vi "Project_G18.vi"() -> ()   [LabVIEW 2022 SP3]
uses:
  <vilib>/DAQmx/read.llb/DAQmx Read (Digital Bool 1Line 1Point).vi
  <vilib>/DAQmx/read.llb/DAQmx Read (Analog 1D DBL NChan 1Samp).vi
  <vilib>/DAQmx/create/channels.llb/DAQmx Create Channel (DI-Digital Input).vi
  <vilib>/DAQmx/create/channels.llb/DAQmx Create Channel (AI-Voltage-Basic).vi
  <vilib>/DAQmx/miscellaneous.llb/DAQmx Fill In Error Info.vi
panel:
  out "BIN STATUS:":string
  out "Dry Waste":bool
  in  "VISA resource name 3":refnum<visa-resource-name>
  in  "Numeric Controller":dbl
  in  "VISA resource name 6":refnum<visa-resource-name>
  out "Object Detector":bool
  in  "Object detector line":tag
  in  "physical channels":tag
  out "Fill level of the bin":u8(slide) scale=0.0..10.0
  out "Wet Waste":bool
  out "Numeric":dbl
  out "Wet/Dry Meter":dbl(knob) scale=0.0..10.0
  in  "Metal detector line":tag
  out "Metal Detector":bool
  in  "VISA resource name 2":refnum<visa-resource-name>
  in  "VISA resource name":refnum<visa-resource-name>
  in  "stop":bool
  # "Smart Waste Management System"
  # "WET"
  # "DRY"
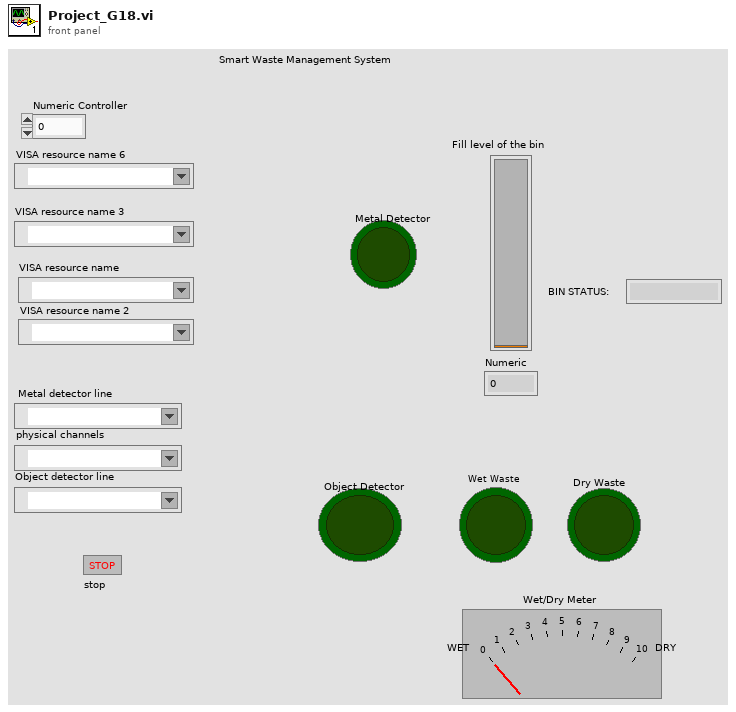
[diagram p1: front panel]
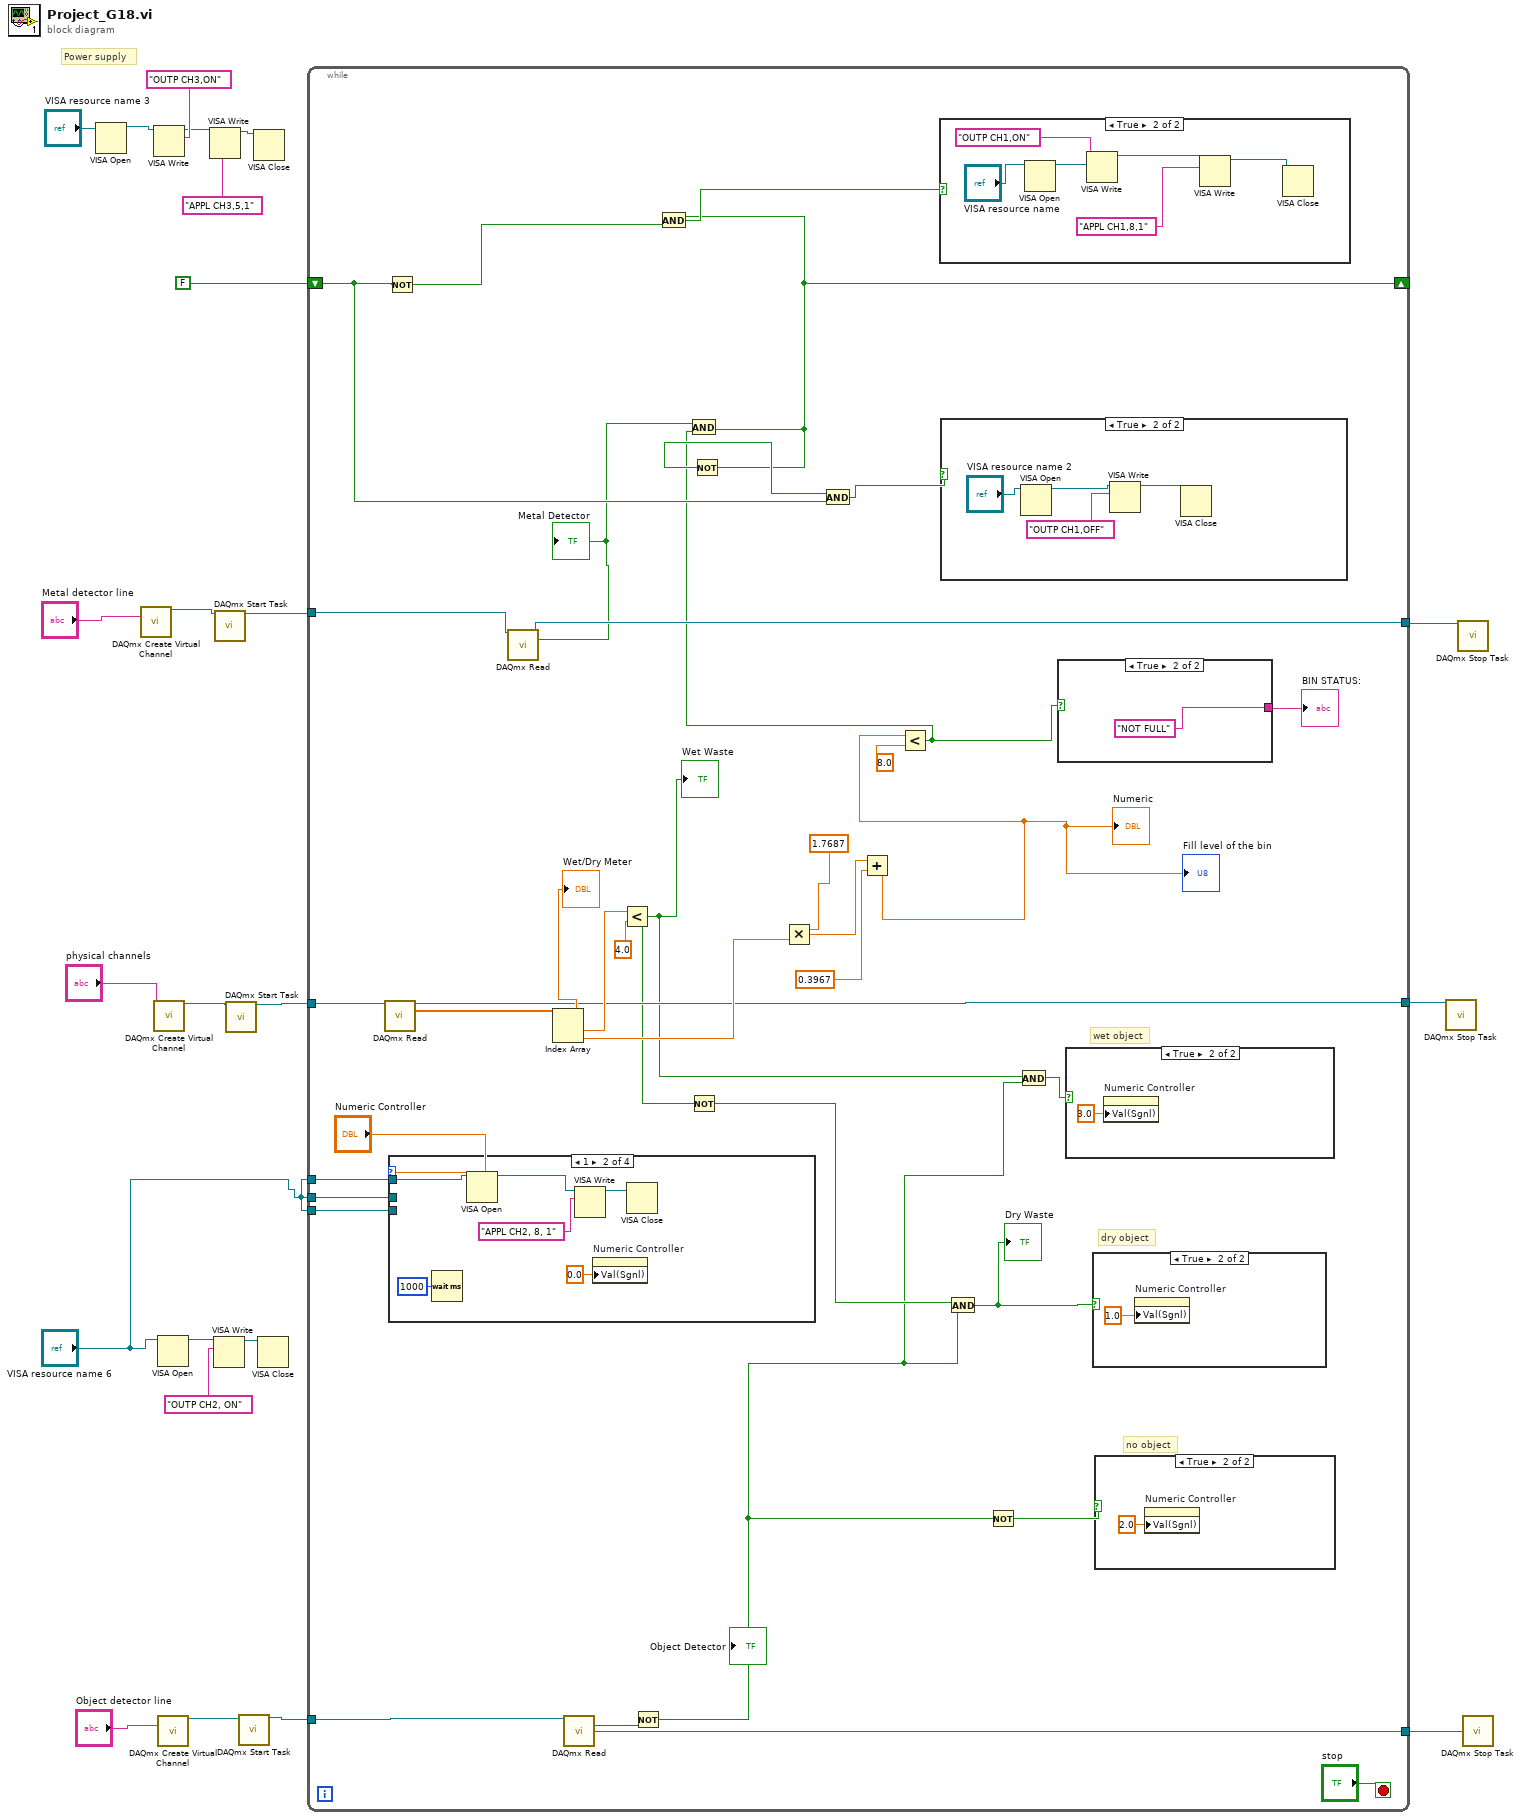
[diagram p0: block diagram]
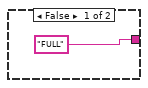
[diagram p2: hidden frame]
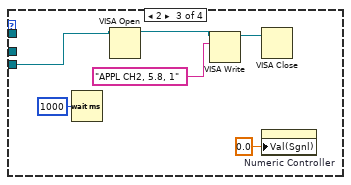
[diagram p7: hidden frame]
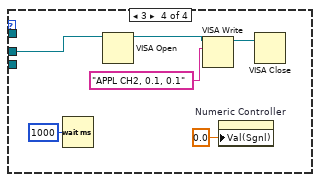
[diagram p8: hidden frame]
diagram:
  # "Power supply"
  n1 = VISA Open(VISA resource name="VISA resource name 3") -> (VISA resource name=w5:refnum<visa-resource-name>)  [unwired: 4 in, 1 out]
  n2 = call-poly <vilib>:"DAQmx Create Virtual Channel.vi"("lines"="Metal detector line") -> ("task out"=w19:refnum<k21>)  [unwired: 13 in, 1 out]
  n3 = VISA Write(VISA resource name=w5, write buffer="OUTP CH3,ON") -> (VISA resource name out=w3:refnum<visa-resource-name>)  [unwired: 1 in, 2 out]
  n4 = call-poly <vilib>:"DAQmx Create Virtual Channel.vi"("physical channels"="physical channels") -> ("task out"=w18:refnum<k21>)  [unwired: 13 in, 1 out]
  n5 = VISA Open(VISA resource name="VISA resource name 6") -> (VISA resource name=w10:refnum<visa-resource-name>)  [unwired: 4 in, 1 out]
  n6 = call-poly <vilib>:"DAQmx Create Virtual Channel.vi"("lines"="Object detector line") -> ("task out"=w14:refnum<k21>)  [unwired: 13 in, 1 out]
  n7 = VISA Write(VISA resource name=w3, write buffer="APPL CH3,5,1") -> (VISA resource name out=w2:refnum<visa-resource-name>)  [unwired: 1 in, 2 out]
  n8 = VISA Write(VISA resource name=w10, write buffer="OUTP CH2, ON") -> (VISA resource name out=w8:refnum<visa-resource-name>)  [unwired: 1 in, 2 out]
  n9 = call <vilib>:"DAQmx Start Task.vi"("task/channels in"=w19) -> ("task out"=w22:refnum<k21>)  [unwired: 13 in, 1 out]
  n10 = call <vilib>:"DAQmx Start Task.vi"("task/channels in"=w18) -> ("task out"=w17:refnum<k21>)  [unwired: 13 in, 1 out]
  n11 = call <vilib>:"DAQmx Start Task.vi"("task/channels in"=w14) -> ("task out"=w13:refnum<k21>)  [unwired: 13 in, 1 out]
  n12 = VISA Close(VISA resource name=w2) -> ()  [unwired: 1 in, 1 out]
  n13 = VISA Close(VISA resource name=w8) -> ()  [unwired: 1 in, 1 out]
  n14 = while {
    shift-right: [w50] -> _
    shift-left: FALSE -> [w56]
    tunnel: w22 -> [w53]
    tunnel: [w52] -> w21
    tunnel: w17 -> [w42]
    tunnel: [w41] -> w15
    tunnel: w13 -> [w40]
    tunnel: [w39] -> w11
    tunnel: "VISA resource name 6" -> [w36]
    tunnel: "VISA resource name 6" -> [w33]
    tunnel: "VISA resource name 6" -> [w29]
    stop <- "stop" stop-if-true
    # "wet object"
    # "no object"
    # "dry object"
    n15 = call-poly <vilib>:"DAQmx Read.vi"("task/channels in"=w42) -> ("task out"=w41:refnum<k21>, "data"=w49:dbl[])  [unwired: 12 in, 1 out]
    n16 = Not(x=w56) -> (.not. x?=w58:bool)
    n17 = case shown="1" "Numeric Controller" {
      tunnel: w36 -> [_ w68 _ _]
      tunnel: w33 -> [_ _ w72 _]
      tunnel: w29 -> [_ _ _ w78]
      frame 0, Default {
      }
      frame 1 {
        n18 = Wait (ms)(milliseconds to wait=u32 1000) -> ()  [unwired: 1 out]
        n19 = VISA Open(VISA resource name=w68) -> (VISA resource name=w69:refnum<visa-resource-name>)  [unwired: 4 in, 1 out]
        n20 = VISA Write(VISA resource name=w69, write buffer="APPL CH2, 8, 1") -> (VISA resource name out=w67:refnum<visa-resource-name>)  [unwired: 1 in, 2 out]
        n21 = property on="Numeric Controller" class="DigNum (strict)"("Val(Sgnl)"=0.0 ("Value (Signaling)")) -> ()  [unwired: 2 in, 2 out]
        n22 = VISA Close(VISA resource name=w67) -> ()  [unwired: 1 in, 1 out]
      }
      frame 2 {
        n23 = Wait (ms)(milliseconds to wait=u32 1000) -> ()  [unwired: 1 out]
        n24 = VISA Open(VISA resource name=w72) -> (VISA resource name=w75:refnum<visa-resource-name>)  [unwired: 4 in, 1 out]
        n25 = VISA Write(VISA resource name=w75, write buffer="APPL CH2, 5.8, 1") -> (VISA resource name out=w74:refnum<visa-resource-name>)  [unwired: 1 in, 2 out]
        n26 = VISA Close(VISA resource name=w74) -> ()  [unwired: 1 in, 1 out]
        n27 = property on="Numeric Controller" class="DigNum (strict)"("Val(Sgnl)"=0.0 ("Value (Signaling)")) -> ()  [unwired: 2 in, 2 out]
      }
      frame 3 {
        n28 = Wait (ms)(milliseconds to wait=u32 1000) -> ()  [unwired: 1 out]
        n29 = VISA Open(VISA resource name=w78) -> (VISA resource name=w81:refnum<visa-resource-name>)  [unwired: 4 in, 1 out]
        n30 = VISA Write(VISA resource name=w81, write buffer="APPL CH2, 0.1, 0.1") -> (VISA resource name out=w80:refnum<visa-resource-name>)  [unwired: 1 in, 2 out]
        n31 = property on="Numeric Controller" class="DigNum (strict)"("Val(Sgnl)"=0.0 ("Value (Signaling)")) -> ()  [unwired: 2 in, 2 out]
        n32 = VISA Close(VISA resource name=w80) -> ()  [unwired: 1 in, 1 out]
      }
    }
    n33 = call-poly <vilib>:"DAQmx Read.vi"("task/channels in"=w53) -> ("task out"=w52:refnum<k21>, "data"=w51:bool)  [unwired: 12 in, 1 out]
    "Metal Detector" <- w51
    n34 = Index Array(array=w49) -> (element #1=w44:dbl, element #2=w45:dbl)  [unwired: 2 in]
    "Wet/Dry Meter" <- w44
    n35 = call-poly <vilib>:"DAQmx Read.vi"("task/channels in"=w40) -> ("task out"=w39:refnum<k21>, "data"=w38:bool)  [unwired: 12 in, 1 out]
    n36 = Less?(x=w44, y=4.0) -> (x < y?=w32:bool)
    "Wet Waste" <- w32
    n37 = Not(x=w38) -> (.not. x?=w30:bool)
    "Object Detector" <- w30
    n38 = Not(x=w32) -> (.not. x?=w35:bool)
    n39 = Multiply(x=1.7687, y=w45) -> (x*y=w47:dbl)
    n40 = Add(x=w47, y=0.3967) -> (x+y=w28:dbl)
    "Numeric" <- w28
    "Fill level of the bin" <- w28
    n41 = Less?(x=w28, y=8.0) -> (x < y?=w25:bool)
    n42 = And(x=w51, y=w25) -> (x .and. y?=w50:bool)
    n43 = And(x=w50, y=w58) -> (x .and. y?=w57:bool)
    n44 = Not(x=w50) -> (.not. x?=w55:bool)
    n45 = And(x=w55, y=w56) -> (x .and. y?=w54:bool)
    n46 = case shown="True" w57 {
      frame False {
      }
      frame True {
        n47 = VISA Open(VISA resource name="VISA resource name") -> (VISA resource name=w92:refnum<visa-resource-name>)  [unwired: 4 in, 1 out]
        n48 = VISA Write(VISA resource name=w92, write buffer="OUTP CH1,ON") -> (VISA resource name out=w91:refnum<visa-resource-name>)  [unwired: 1 in, 2 out]
        n49 = VISA Write(VISA resource name=w91, write buffer="APPL CH1,8,1") -> (VISA resource name out=w90:refnum<visa-resource-name>)  [unwired: 1 in, 2 out]
        n50 = VISA Close(VISA resource name=w90) -> ()  [unwired: 1 in, 1 out]
      }
    }
    n51 = case shown="True" w54 {
      frame False {
      }
      frame True {
        n52 = VISA Open(VISA resource name="VISA resource name 2") -> (VISA resource name=w86:refnum<visa-resource-name>)  [unwired: 4 in, 1 out]
        n53 = VISA Write(VISA resource name=w86, write buffer="OUTP CH1,OFF") -> (VISA resource name out=w85:refnum<visa-resource-name>)  [unwired: 1 in, 2 out]
        n54 = VISA Close(VISA resource name=w85) -> ()  [unwired: 1 in, 1 out]
      }
    }
    n55 = And(x=w35, y=w30) -> (x .and. y?=w26:bool)
    "Dry Waste" <- w26
    n56 = Not(x=w30) -> (.not. x?=w34:bool)
    n57 = And(x=w32, y=w30) -> (x .and. y?=w31:bool)
    n58 = case shown="True" w25 {
      tunnel: ["FULL" ("BIN Status:") "NOT FULL" ("BIN Status:")] -> w24
      frame False {
      }
      frame True {
      }
    }
    "BIN STATUS:" <- w24
    n59 = case shown="True" w31 {
      frame False {
      }
      frame True {
        n60 = property on="Numeric Controller" class="DigNum (strict)"("Val(Sgnl)"=3.0 ("Value (Signaling)")) -> ()  [unwired: 2 in, 2 out]
      }
    }
    n61 = case shown="True" w26 {
      frame False {
      }
      frame True {
        n62 = property on="Numeric Controller" class="DigNum (strict)"("Val(Sgnl)"=1.0 ("Numeric 2")) -> ()  [unwired: 2 in, 2 out]
      }
    }
    n63 = case shown="True" w34 {
      frame False {
      }
      frame True {
        n64 = property on="Numeric Controller" class="DigNum (strict)"("Val(Sgnl)"=2.0 ("Value (Signaling)")) -> ()  [unwired: 2 in, 2 out]
      }
    }
  }
  n65 = call <vilib>:"DAQmx Stop Task.vi"("task/channels in"=w15) -> ()  [unwired: 13 in, 2 out]
  n66 = call <vilib>:"DAQmx Stop Task.vi"("task/channels in"=w21) -> ()  [unwired: 13 in, 2 out]
  n67 = call <vilib>:"DAQmx Stop Task.vi"("task/channels in"=w11) -> ()  [unwired: 13 in, 2 out]
